vi "Initialize.vi"(8 "error in":errorcluster, 9 "Path":path, 10 "Device":string, 11 "Chronometer in":refnum<class "Chronometer.lvclass">) -> (0 "error out":errorcluster, 3 "Chronometer out":refnum<class "Chronometer.lvclass">)   [LabVIEW 2023, in "Chronometer.lvlib" / "Chronometer.lvclass"]
uses:
  Chronometer.lvclass
  builds/Tools/Config.lvlibp/Config.lvclass
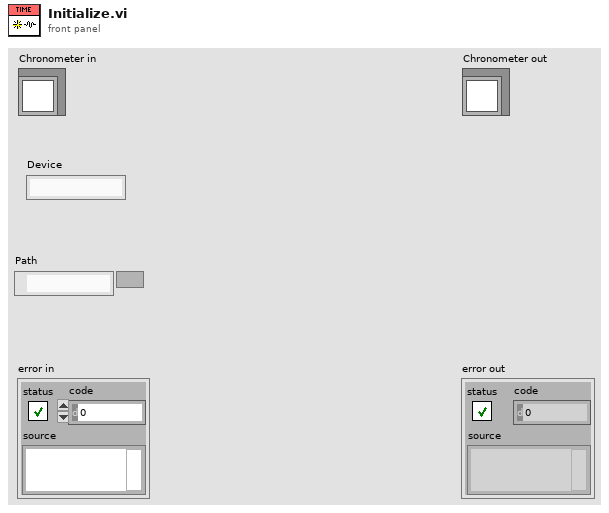
[diagram p1: front panel]
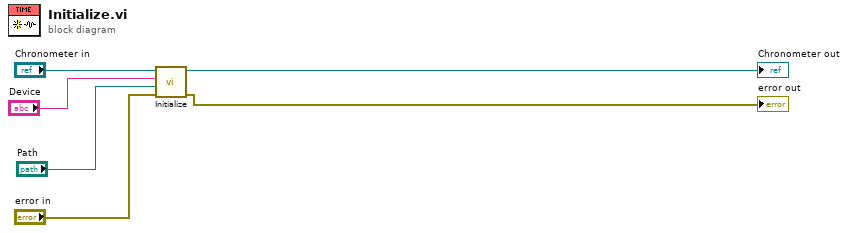
[diagram p0: block diagram]
diagram:
  n1 = call-parent "Initialize.vi"("error in"="error in", "Path"="Path", "Device"="Device", "Config in"="Chronometer in") -> ("error out"=→"error out":errorcluster, "Config out"=→"Chronometer out":refnum<class "Chronometer.lvclass">)  [unwired: 6 in]
